vi "Test Compute Text Size.vi"(8 "error in (no error)":errorcluster, 11 "Test Case In":refnum<class "01_Image.lvclass">) -> (0 "error out":errorcluster, 3 "Test Case Out":refnum<class "01_Image.lvclass">)   [LabVIEW 2020, in "test.lvlib" / "01_Image.lvclass"]
uses:
  01_Image.lvclass
  C:/Program Files (x86)/National Instruments/LabVIEW 2026/vi.lib/Astemes/LUnit/Test Case.lvclass
  image/Text Drawing Settings.ctl
  image/Font Face.ctl
  common/Image Size (Integer).ctl
  <vilib>/Astemes/LUnit/Test Case.lvclass/Test Case.ctl
  4993e8ee-a06a-463a-9684-69129f64d5ce.vi
  image/Required Font-Scale (As Numeric).vi
  <vilib>/Astemes/LUnit/Core/LUnit Test Case/Private/Append Pass Result.vi
  <vilib>/Astemes/LUnit/Core/LUnit Test Case/Private/Append Fail Result.vi
  4993e8ee-a06a-463a-9684-69129f64d5ce.vi/9c5d11cd-9439-4240-a1ee-d9baace9c924.vi
  <vilib>/Astemes/LUnit/Core/LUnit Test Case/Private/Run In UI.vi
  <vilib>/Utility/error.llb/Clear Errors.vi
  <vilib>/Utility/error.llb/Error Cluster From Error Code.vi
  image/image.lvlib
  common/common.lvlib
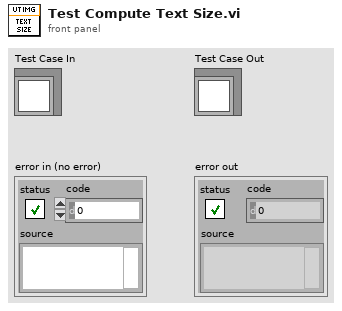
[diagram p1: front panel]
types:
  T1 = typedef "common.lvlib/Image Size (Integer).ctl" = cluster{"Width":u16, "Height":u16}
  T2 = typedef "image.lvlib/Text Drawing Settings.ctl" = cluster{"OpenCV Font Face":T3, "Font Scale":dbl}
  T3 = typedef "image.lvlib/Font Face.ctl" = enum8{"FONT_HERSHEY_SIMPLEX", "FONT_HERSHEY_PLAIN", "FONT_HERSHEY_DUPLEX", "FONT_HERSHEY_COMPLEX", "FONT_HERSHEY_TRIPLEX", "FONT_HERSHEY_COMPLEX_SMALL", "FONT_HERSHEY_SCRIPT_SIMPLEX", "FONT_HERSHEY_SCRIPT_COMPLEX", "FONT_ITALIC"}
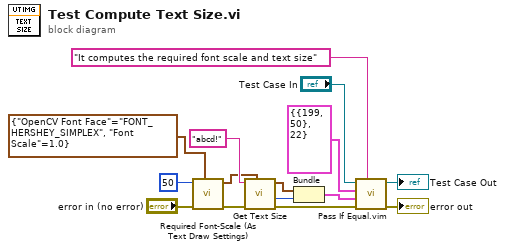
[diagram p0: block diagram]
diagram:
  n1 = call "Required Font-Scale (As Text Draw Settings).vi"("Text Drawing Settings in (Default: Simplex)"=T2 {"OpenCV Font Face"=enum."FONT_HERSHEY_SIMPLEX", "Font Scale"=1.0} ("Text Drawing Settings (Default: Simplex, Top-Left)"), "error in (no error)"="error in (no error)", "Required Text Height"=u16 50) -> ("error out"=w12:errorcluster, "Text Drawing Settings out"=w1:T2)  [unwired: 7 in]
  n2 = call "Get Text Size.vi"("Text Drawing Settings (Default: Simplex)"=w1, "error in (no error)"=w12, "Text"="abcd!") -> ("error out"=w3:errorcluster, "Base Line"=w7:i32, "Size"=w8:T1)  [unwired: 6 in]
  n3 = Bundle("Size"=w8, "Base Line"=w7) -> (w4:cluster{"Size":T1, "Base Line":i32})  [unwired: 1 in]
  n4 = call "Pass If Equal.vim"("Description"="It computes the required font scale and text size", "error in (no error)"=w3, "Actual"=w4, "Expected"=cluster{"Size":T1, "Base Line":i32} {"Size"={"Width"=199, "Height"=50}, "Base Line"=22}, "LUnit Test Case In"="Test Case In") -> ("error out"=→"error out":errorcluster, "LUnit Test Case Out"=→"Test Case Out":refnum<class "01_Image.lvclass">)  [unwired: 5 in]
